vi "sort_2D_array_by_x.vi"(11 "arrays":cluster{dbl[], dbl[]}) -> (2 "X out":dbl[](array[numeric]), 3 "Y out":dbl[](array[numeric]))   [LabVIEW 2015]
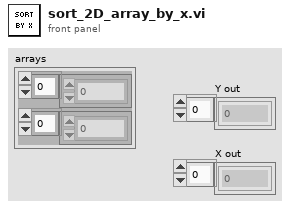
[diagram p1: front panel]
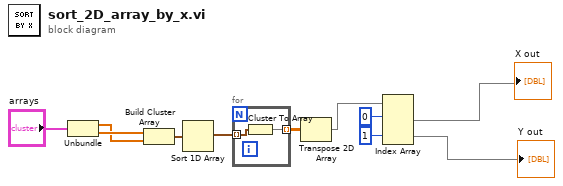
[diagram p0: block diagram]
diagram:
  n1 = Unbundle("arrays") -> (w1:dbl[], w2:dbl[])
  n2 = Build Cluster Array(w2, w1) -> (w4:cluster{"element":dbl, "element":dbl}[])
  n3 = Sort 1D Array(array=w4) -> (sorted array=w5:cluster{"element":dbl, "element":dbl}[])
  n4 = for {
    tunnel: w5 -> [w13] mode=indexing
    tunnel: [w12] -> w8 mode=indexing
    n5 = Cluster To Array(cluster=w13) -> (array=w12:dbl[])
  }
  n6 = Transpose 2D Array(2D array=w8) -> (transposed array=w9:dbl[][])
  n7 = Index Array(array=w9, index (row) #1=0 ("index (row)"), index (row) #2=1 ("index (row)")) -> (element #1=→"X out":dbl[], element #2=→"Y out":dbl[])  [unwired: 2 in]
